vi "setTitle.vi"(9 "Title":string, 11 "String in":string) -> (1 "command":string, 3 "String out":string)   [LabVIEW 2012]
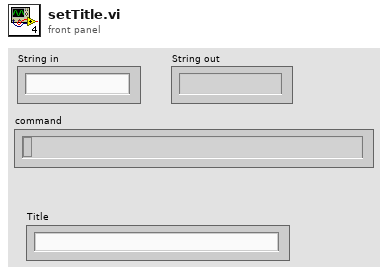
[diagram p1: front panel]
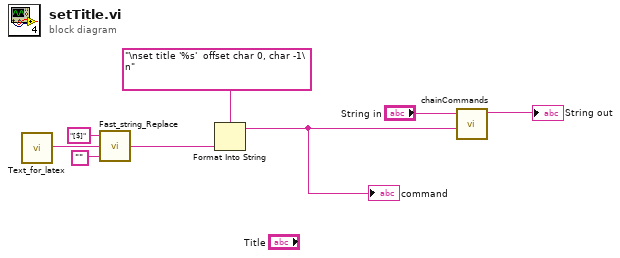
[diagram p0: block diagram]
diagram:
  n1 = call "Text_for_latex.vi"() -> ("Output String"=w7:string)  [unwired: 1 in]
  n2 = call "Fast_string_Replace.vi"("Replace match with:"="", "Input String"=w7, "regular expression"="[$]") -> ("Output String"=w8:string)  [unwired: 2 out]
  n3 = Format Into String(format string="\nset title '%s'  offset char 0, char -1\n", w8) -> (resulting string=w2:string)  [unwired: 2 in, 1 out]
  "command" <- w2
  n4 = call "chainCommands.vi"("Command"=w2, "String in"="String in") -> ("String 2"=→"String out":string)  [unwired: 9 in]
